vi "Condition Msg Init Msg VI.vi"(8 "error in":errorcluster, 9 "Msg All Terminals":i32[](array[numeric]), 10 "Name Msg Refs.Init Msg VI":refnum<vi>) -> (0 "error out":errorcluster)   [LabVIEW 2025, in "_Rescript.lvlib" / "Msg.lvlib" / "Msg.lvclass"]
uses:
  <vilib>/Utility/traverseref.llb/TRef TravTarget.ctl
  Msg.lvclass
  Msg.lvclass/Msg.ctl
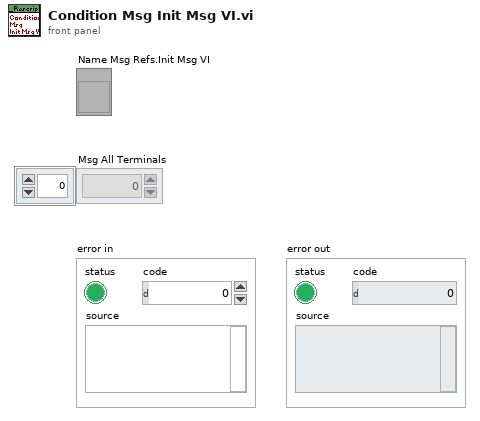
[diagram p1: front panel]
types:
  T1 = typedef "TRef TravTarget.ctl" = enum16{"FP", "BD", "Other"}
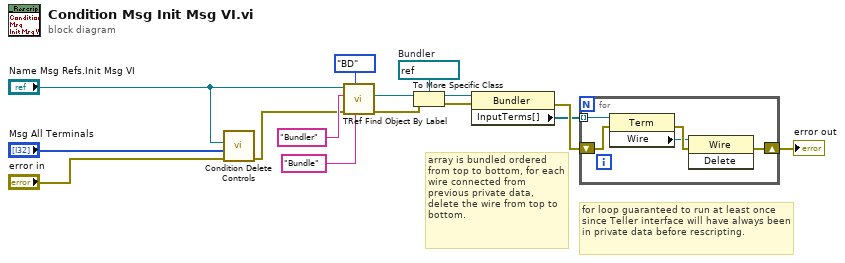
[diagram p0: block diagram]
diagram:
  w12 = refnum<vi> refnum  # Bundler
  # "array is bundled ordered from top to bottom, for each wire connected from previous private data, delete the wire from top to bottom."
  # "for loop guaranteed to run at least once since Teller interface will have always been in private data before rescripting."
  n1 = call "Condition Delete Controls.vi"("error in"="error in", "Terminals"="Msg All Terminals", "VI"="Name Msg Refs.Init Msg VI") -> ("error out"=w3:errorcluster)  [unwired: 8 in]
  n2 = call <vilib>:"TRef Find Object By Label.vi"("Label"="Bundle", "Traverse Target"=TRef_TravTarget."BD", "error in (no error)"=w3, "Class Name"="Bundler", "VI Ref"="Name Msg Refs.Init Msg VI") -> ("error out"=w13:errorcluster, "Found Obj Ref"=w11:refnum<vi>)  [unwired: 3 in, 2 out]
  n3 = To More Specific Class(target class=w12, reference=w11, error in=w13) -> (specific class reference=w8:refnum<vi>, error out=w6:errorcluster)
  n4 = property class="Bundler"(reference=w8, error in=w6) -> (error out=w14:errorcluster, "InputTerms[]"=w5:refnum<vi>[])  [unwired: 1 out]
  n5 = for {
    shift-right: [w16] -> w4
    shift-left: w14 -> [w17]
    tunnel: w5 -> [w19] mode=indexing
    n6 = property class="Term"(reference=w19, error in=w17) -> (error out=w20:errorcluster, "Wire"=w18:refnum<vi>)  [unwired: 1 out]
    n7 = invoke class="Wire" method="Delete"(reference=w18, error in=w20) -> (error out=w16:errorcluster)  [unwired: 1 in, 2 out]
  }
  "error out" <- w4
